vi "Configure from DBC.vi"(8 "error in":errorcluster, 11 "PCAN in":refnum<class "PCAN.lvclass">) -> (0 "error out":errorcluster, 3 "PCAN out":refnum<class "PCAN.lvclass">)   [LabVIEW 2023, in "PCAN.lvclass"]
uses:
  PCAN.lvclass
  D:/git/HAL/HAL/Configurations/CFG JSON/CFG JSON.lvclass
  PCAN.lvclass/PCAN.ctl
  e876bc77-3914-497d-9dbf-46d43ff41845.vi
  e876bc77-3914-497d-9dbf-46d43ff41845.vi/a4169a97-72fc-4003-a778-603cf20cafa0.vi
  <vilib>/JDP Science/JSONtext/Find Item.vi
  <vilib>/JDP Science/JSONtext/Next JSON Value.vi
  <vilib>/JDP Science/JSONtext/String Subset.vi
  <vilib>/JDP Science/JSONtext/Parsing/Advance past next JSON Value (inlined COPY).vi
  <vilib>/JDP Science/JSONtext/Parsing/Advance past whitespace.vi
  <vilib>/JDP Science/JSONtext/Parsing/Advance past String.vi
  <vilib>/JDP Science/JSONtext/Parsing/Advance past Number.vi
  <vilib>/JDP Science/JSONtext/Parsing/Advance past Line Ending.vi
  <vilib>/JDP Science/JSONtext/Parsing/Parse Full Path or Item Name.vi
  <vilib>/JDP Science/JSONtext/Parsing/Advance past Array.vi
  <vilib>/JDP Science/JSONtext/Parsing/Advance past Object.vi
  <vilib>/JDP Science/JSONtext/support/Error Cluster From Code.vi
  <vilib>/JDP Science/JSONtext/Offset/Find Item Locations by Path.vi
  <vilib>/JDP Science/JSONtext/JSON text to Variant.vi
  <userlib>/_OpenG.lib/file/file.llb/File Exists - Scalar__ogtk.vi
  <vilib>/JDP Science/JSONtext/LVClass Serializer/JSONtext LVClass Serializer.lvclass
  <vilib>/xnet/xnet.llb/XNET Create Session (Conversion).vi
  <resource>/objmgr/xnet.rc
  Configurations/CFG JSON/CFG JSON.lvclass
  <userlib>/_OpenG.lib/file/file.llb/openg_file.lvlib
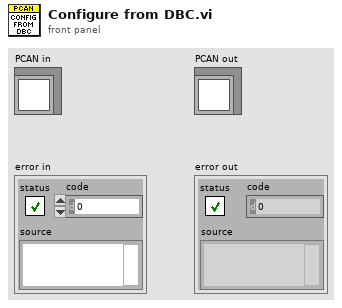
[diagram p1: front panel]
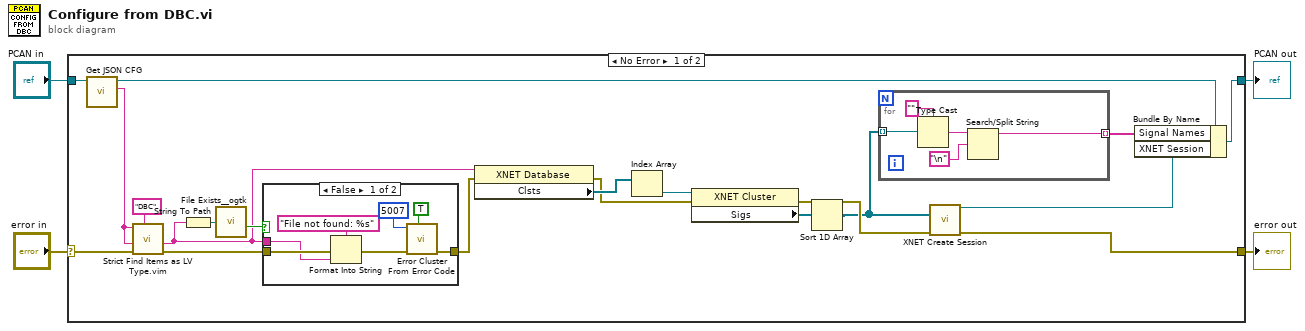
[diagram p0: block diagram]
diagram:
  n1 = case shown="No Error" "error in" {
    selector: "error in" -> [w23 w39]
    tunnel: [w12 w39] -> w3
    tunnel: [w21 w38] -> w1
    tunnel: "PCAN in" -> [w24 w38]
    frame No Error {
      n2 = call "Get JSON CFG.vi"("CFG JSON in"=w24) -> ("<JSON> CFG"=w19:string, "CFG JSON out"=w16:refnum<class "PCAN.lvclass">)  [unwired: 9 in]
      n3 = call "Strict Find Items as LV Type.vim"("$Path or Item Name"="DBC", "error in"=w23, "Data Type and Default Value"=w19, "<JSON>"=w19) -> ("error out"=w8:errorcluster, "Data out"=w7:string)  [unwired: 5 in, 1 out]
      n4 = String To Path(string=w7) -> (path=w5:path)
      n5 = call-poly <userlib>:"File Exists__ogtk.vi"("file path"=w5) -> ("exists"=w9:bool)  [unwired: 6 in, 1 out]
      n6 = case shown="False" w9 {
        tunnel: w8 -> [w27 w32]
        tunnel: w7 -> [w25 _]
        tunnel: [w30 w32] -> w6
        frame False {
          n7 = Format Into String(format string="File not found: %s", error in=w27, w25) -> (error out=w28:errorcluster)  [unwired: 1 in, 1 out]
          n8 = call <vilib>:"Error Cluster From Error Code.vi"("show call chain? (False)"=TRUE, "error in (no error)"=w28, "error code (0)"=5007) -> ("error out"=w30:errorcluster)  [unwired: 6 in]
        }
        frame True {
        }
      }
      n9 = property class="XNET Database"(reference=w7, error in=w6) -> (error out=w18:errorcluster, "Clsts"=w22:refnum<k21>[])  [unwired: 1 out]
      n10 = Index Array(array=w22) -> (element=w14:refnum<k21>)  [unwired: 1 in]
      n11 = property class="XNET Cluster"(reference=w14, error in=w18) -> (error out=w13:errorcluster, "Sigs"=w11:refnum<k21>[])  [unwired: 1 out]
      n12 = Sort 1D Array(array=w11) -> (sorted array=w10:refnum<k21>[])
      n13 = for {
        tunnel: w10 -> [w37] mode=indexing
        tunnel: [w34] -> w15 mode=indexing
        n14 = Type Cast(type="", x=w37) -> (*(type *) &x=w35:string)
        n15 = Search/Split String(string=w35, search string/char (-)="\n") -> (substring before match=w34:string)  [unwired: 1 in, 2 out]
      }
      n16 = call-poly <vilib>:"XNET Create Session.vi"("signal list"=w10, "error in (no error)"=w13) -> ("session out"=w17:refnum<k21>, "error out"=w12:errorcluster)  [unwired: 12 in]
      n17 = Bundle By Name(cluster=w16, "Signal Names"=w15, "XNET Session"=w17) -> (w21:refnum<class "PCAN.lvclass">)
    }
    frame Error {
    }
  }
  "error out" <- w3
  "PCAN out" <- w1
